vi "Cut over Item Sym.vi"(6 "Position":T1, 8 "error in (no error)":errorcluster, 9 "MulticolumnListbox in":refnum<vi>) -> (0 "error out":errorcluster)   [LabVIEW 2017]
uses:
  <vilib>/Utility/miscctls.llb/LVPositionTypeDef.ctl
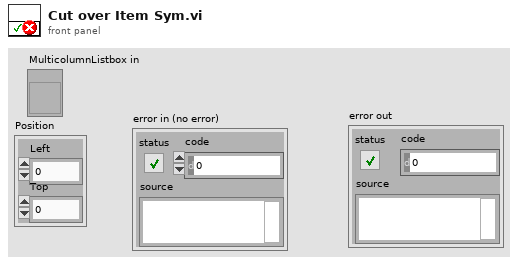
[diagram p1: front panel]
types:
  T1 = typedef "LVPositionTypeDef.ctl" = cluster{"Left":i32, "Top":i32}
  T2 = typedef "LVRowAndColumnTypeDef.ctl" = cluster{"Row":i32, "Column":i32}
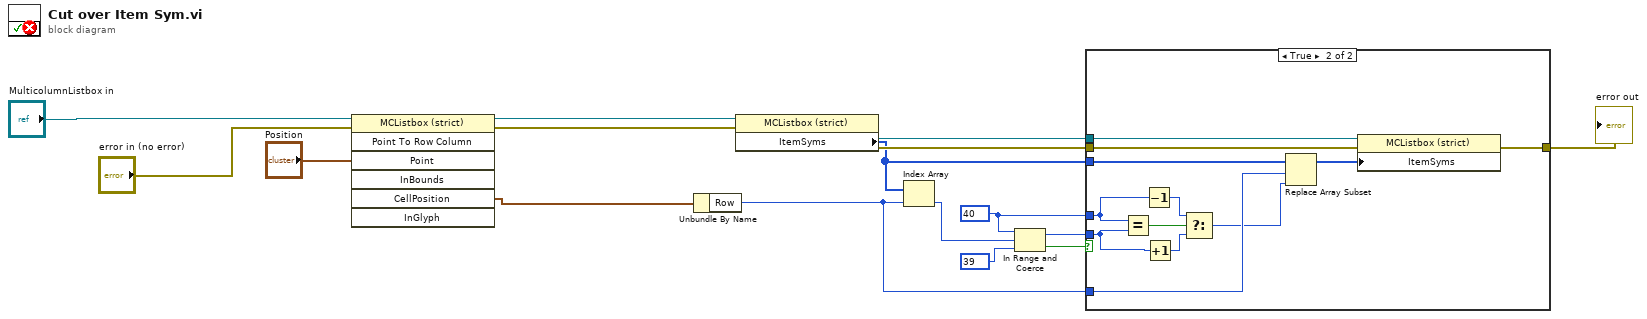
[diagram p0: block diagram]
diagram:
  w12 = 40
  n1 = invoke class="MCListbox (strict)" method="Point To Row Column"(reference="MulticolumnListbox in", error in="error in (no error)", "Point"="Position") -> (reference out=w6:refnum<vi>, error out=w5:errorcluster, "CellPosition"=w4:T2)  [unwired: 4 in, 4 out]
  n2 = Unbundle By Name(w4) -> ("Row"=w8:i32)
  n3 = property class="MCListbox (strict)"(reference=w6, error in=w5) -> (reference out=w11:refnum<vi>, error out=w10:errorcluster, "ItemSyms"=w9:i32[])
  n4 = Index Array(array=w9, index=w8) -> (element=w15:i32)
  n5 = In Range and Coerce(upper limit=w12, x=w15, lower limit=39) -> (coerced(x)=w13:i32, In Range?=w14:bool)
  n6 = case shown="True" w14 {
    tunnel: w13 -> [_ w26]
    tunnel: w12 -> [_ w27]
    tunnel: w11 -> [_ w21]
    tunnel: w10 -> [w17 w20]
    tunnel: w9 -> [_ w24]
    tunnel: w8 -> [_ w23]
    tunnel: [w17 w18] -> w7
    frame False {
    }
    frame True {
      n7 = Equal?(x=w27, y=w26) -> (x = y?=w29:bool)
      n8 = Decrement(x=w27) -> (x-1=w28:i32)
      n9 = Increment(x=w26) -> (x+1=w25:i32)
      n10 = Select(t=w28, s=w29, f=w25) -> (s? t:f=w22:i32)
      n11 = Replace Array Subset(array=w24, new element=w22, index=w23) -> (w19:i32[])
      n12 = property class="MCListbox (strict)"(reference=w21, error in=w20, "ItemSyms"=w19) -> (error out=w18:errorcluster)  [unwired: 1 out]
    }
  }
  "error out" <- w7
